vi "Read_Routing_Data.vi"(7 "table":string, 8 "error in (no error)":errorcluster, 11 "Ref In":T1={"MS SQL Connection"=refnum, "UDL File"=path "", "Time"="", "DCODE"="", "WIP+1"=0, "MC No?"=0, "POKAYOKE?"=FALSE, "Expected Result"="", "Result [Status]"="", "Clock"=0.0, "RFID"="", "WIP Queue"=refnum, "TS Parameter"={"ProfitCenterCode"="", "LineCode"="", "WorkOrderNumber"="", "Model"="", "Model_with_Prefix"="", "VendorCode"="", "SetParameterDateCode"="", "PokaYoke"=0, "Target"=1, "Live_DateCode"="", "CustomerPartNumber"="", "Hand"="", "sBarcode"=FALSE, "FCA"=0, "Ent_Stamp"=timestamp(0 s since 1904-01-01), "STS_CD"=0.0}, "Data_Queue"=[], "RFID Serial No."=""} {"TS Parameter"."FCA" format="%01d"; "TS Parameter"."Target" min=1 max=100000; "TS Parameter"."PokaYoke" min=0 max=1}) -> (0 "error out":errorcluster, 2 "Routing Data":T4[](array[typedef]), 3 "Ref Out":T1={"MS SQL Connection"=refnum, "UDL File"=path "", "Time"="", "DCODE"="", "WIP+1"=0, "MC No?"=0, "POKAYOKE?"=FALSE, "Expected Result"="", "Result [Status]"="", "Clock"=0.0, "RFID"="", "WIP Queue"=refnum, "TS Parameter"={"ProfitCenterCode"="", "LineCode"="", "WorkOrderNumber"="", "Model"="", "Model_with_Prefix"="", "VendorCode"="", "SetParameterDateCode"="", "PokaYoke"=0, "Target"=1, "Live_DateCode"="", "CustomerPartNumber"="", "Hand"="", "sBarcode"=FALSE, "FCA"=0, "Ent_Stamp"=timestamp(0 s since 1904-01-01), "STS_CD"=0.0}, "Data_Queue"=[], "RFID Serial No."=""} {"TS Parameter"."FCA" format="%01d"; "TS Parameter"."Target" min=1 max=100000; "TS Parameter"."PokaYoke" min=0 max=1})   [LabVIEW 2020]
uses:
  Controls/TD SQL.ctl
  <vilib>/addons/database/Connection.llb/Conn ObjectReference.ctl
  Controls/WIP_State.ctl
  Controls/TS_Parameter.ctl
  Controls/Routing.ctl
  <menus>/Controls/Devaseelan Style/ONOFF Small.ctl
  <vilib>/regexp/Match Regular Expression.xnode
  <vilib>/addons/database/NI_Database_API.lvlib
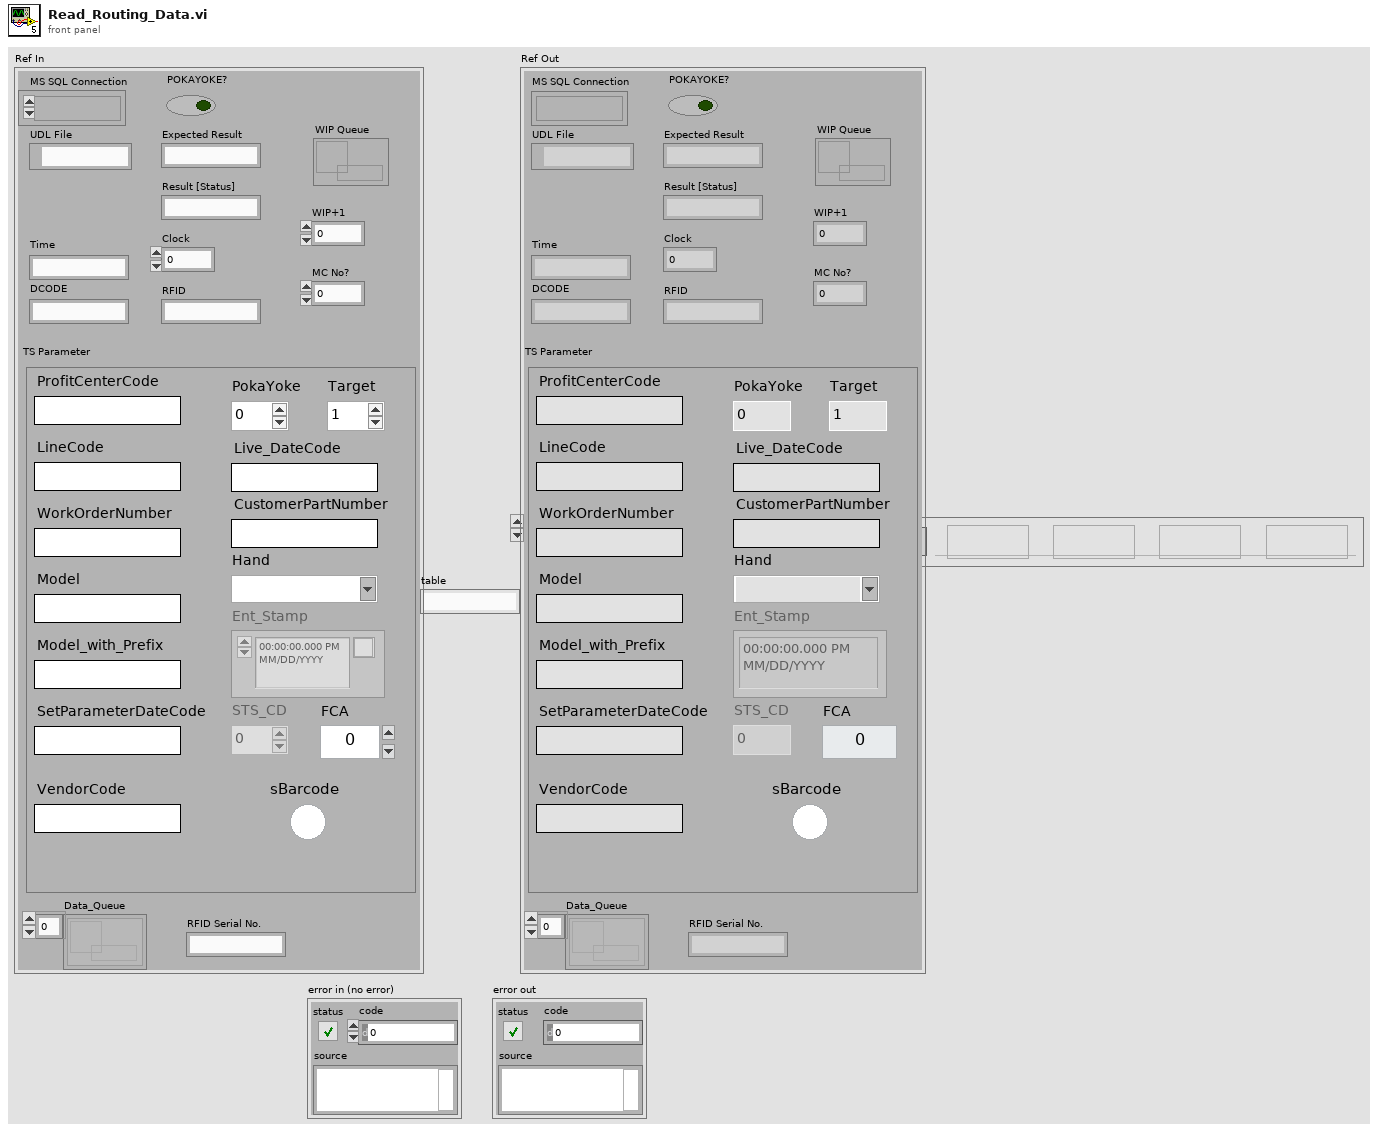
[diagram p1: front panel]
types:
  T1 = typedef "TD SQL.ctl" = cluster{"MS SQL Connection":T2, "UDL File":path, "Time":string, "DCODE":string, "WIP+1":i64, "MC No?":i32, "POKAYOKE?":bool, "Expected Result":string, "Result [Status]":string, "Clock":dbl, "RFID":string, "WIP Queue":refnum<queue>, "TS Parameter":T3, "Data_Queue":refnum<queue>[], "RFID Serial No.":string}
  T2 = typedef "NI_Database_API.lvlib/Conn ObjectReference.ctl" = refnum<k1>
  T3 = typedef "TS_Parameter.ctl" = cluster{"ProfitCenterCode":string, "LineCode":string, "WorkOrderNumber":string, "Model":string, "Model_with_Prefix":string, "VendorCode":string, "SetParameterDateCode":string, "PokaYoke":i32, "Target":i32, "Live_DateCode":string, "CustomerPartNumber":string, "Hand":string, "sBarcode":bool, "FCA":i32, "Ent_Stamp":timestamp, "STS_CD":dbl}
  T4 = typedef "Routing.ctl" = cluster{"OperationSeqNo":i32, "Table Code":string, "OperationCode":string, "MachineCode":string, "OperationRequired":T5, "Traceability":T5, "POKA_YOKE_ALLOWED":T5, "Engraving":T5}
  T5 = typedef "ONOFF Small.ctl" = bool
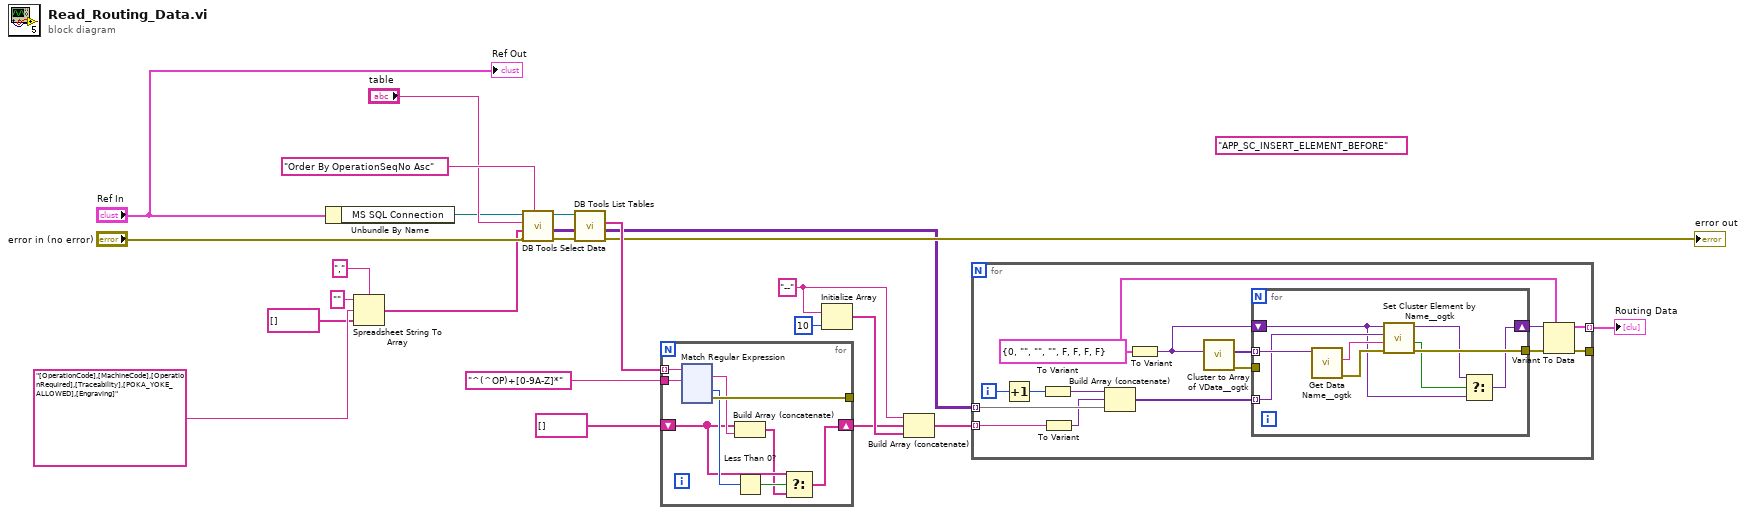
[diagram p0: block diagram]
diagram:
  w20 = "--" ("String")
  (unwired) "APP_SC_INSERT_ELEMENT_BEFORE" ("ItemPath 3")
  n1 = Unbundle By Name("Ref In") -> ("MS SQL Connection"=w2:T2)
  n2 = Spreadsheet String To Array(delimiter (Tab)=",", format string="", spreadsheet string="[OperationCode],[MachineCode],[OperationRequired],[Traceability],[POKA_YOKE_ALLOWED],[Engraving]" ("table"), array type (2D Dbl)=string[] []) -> (array=w8:string[])
  n3 = call <vilib>:"DB Tools Select Data.vi"("condition"="Order By OperationSeqNo Asc" ("table"), "error in (no error)"="error in (no error)", "columns"=w8, "table"="table", "connection reference"=w2) -> ("error out"=w15:errorcluster, "data"=w9:variant[][], "connection reference out"=w11:T2)  [unwired: 1 in]
  n4 = call <vilib>:"DB Tools List Tables.vi"("error in (no error)"=w15, "connection reference"=w11) -> ("error out"=→"error out":errorcluster, "tables"=w17:string[])  [unwired: 3 in, 1 out]
  n5 = for {
    tunnel: "^(^OP)+[0-9A-Z]*" ("String") -> [w32]
    tunnel: w17 -> [w31] mode=indexing
    tunnel: [w30] -> _
    shift-right: [w24] -> w18
    shift-left: string[] [] ("tables") -> [w26]
    n6 = xnode "Match Regular Expression"("input string"=w31, "regular expression"=w32) -> ("whole match"=w28:string, "offset past match"=w29:i32, "error out"=w30:errorcluster)  [unwired: 4 in, 2 out]
    n7 = Build Array (concatenate)(w26, w28) -> (w25:string[])
    n8 = Less Than 0?(x=w29) -> (x < 0?=w27:bool)
    n9 = Select(t=w26, s=w27, f=w25) -> (s? t:f=w24:string[])
  }
  n10 = Initialize Array(w20, 10 ("dimension size")) -> (w22:string[])
  n11 = Build Array (concatenate)(w20, w18, w22) -> (w19:string[])
  n12 = for {
    tunnel: w9 -> [w159] mode=indexing
    tunnel: [w155] -> _
    tunnel: [w154] -> w10 mode=indexing
    tunnel: w19 -> [w149] mode=indexing
    i -> [w153]
    w157 = T4 {"OperationSeqNo"=0, "Table Code"="", "OperationCode"="", "MachineCode"="", "OperationRequired"=FALSE, "Traceability"=FALSE, "POKA_YOKE_ALLOWED"=FALSE, "Engraving"=FALSE} ("Data")
    n13 = Increment(x=w153) -> (x+1=w152:i32)
    n14 = To Variant(anything=w152) -> (Variant=w150:variant)
    n15 = To Variant(anything=w149) -> (Variant=w148:variant)
    n16 = Build Array (concatenate)(w150, w148, w159) -> (w151:variant[])
    n17 = To Variant(anything=w157) -> (Variant=w160:variant)
    n18 = call <userlib>:"Cluster to Array of VData__ogtk.vi"("Cluster"=w160) -> ("error out"=w147:errorcluster, "Array of VData"=w161:variant[])  [unwired: 9 in]
    n19 = for {
      tunnel: w151 -> [w168] mode=indexing
      tunnel: w161 -> [w170] mode=indexing
      shift-right: [w162] -> w158
      shift-left: w160 -> [w163]
      tunnel: [w167] -> w156
      tunnel: w147 -> [_]
      n20 = call <userlib>:"Get Data Name__ogtk.vi"("Data"=w170) -> ("error out"=w166:errorcluster, "Data Name"=w169:string)  [unwired: 8 in, 1 out]
      n21 = call <userlib>:"Set Cluster Element by Name__ogtk.vi"("error in (no error)"=w166, "Element Name (\"\": New Element Data Name)"=w169, "New Element Value"=w168, "Cluster"=w163) -> ("error out"=w167:errorcluster, "found?"=w165:bool, "VCluster out"=w164:variant)  [unwired: 5 in]
      n22 = Select(t=w164, s=w165, f=w163) -> (s? t:f=w162:variant)
    }
    n23 = Variant To Data(error in=w156, type=w157, Variant=w158) -> (data=w154:T4, error out=w155:errorcluster)
  }
  "Routing Data" <- w10
  "Ref Out" <- "Ref In"
